vi "Graph-Init.vi"(8 "error in (no error)":errorcluster, 9 "SR830 in":refnum<vi>, 10 "Parameters":refnum<vi>, 11 "WaveformChart in":refnum<vi>) -> (0 "error out":errorcluster)   [LabVIEW 2016]
uses:
  controls/Parameters.ctl
  controls/Lambda.ctl
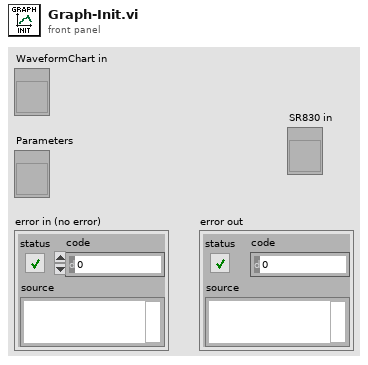
[diagram p1: front panel]
types:
  T1 = typedef "Parameters.ctl" = cluster{"Lambda":T2, "Power":dbl, "Frequency":dbl, "Stabilizing":dbl, "Samples":dbl, "File":path}
  T2 = typedef "Lambda.ctl" = cluster{"Init":dbl, "Final":dbl, "dx":dbl}
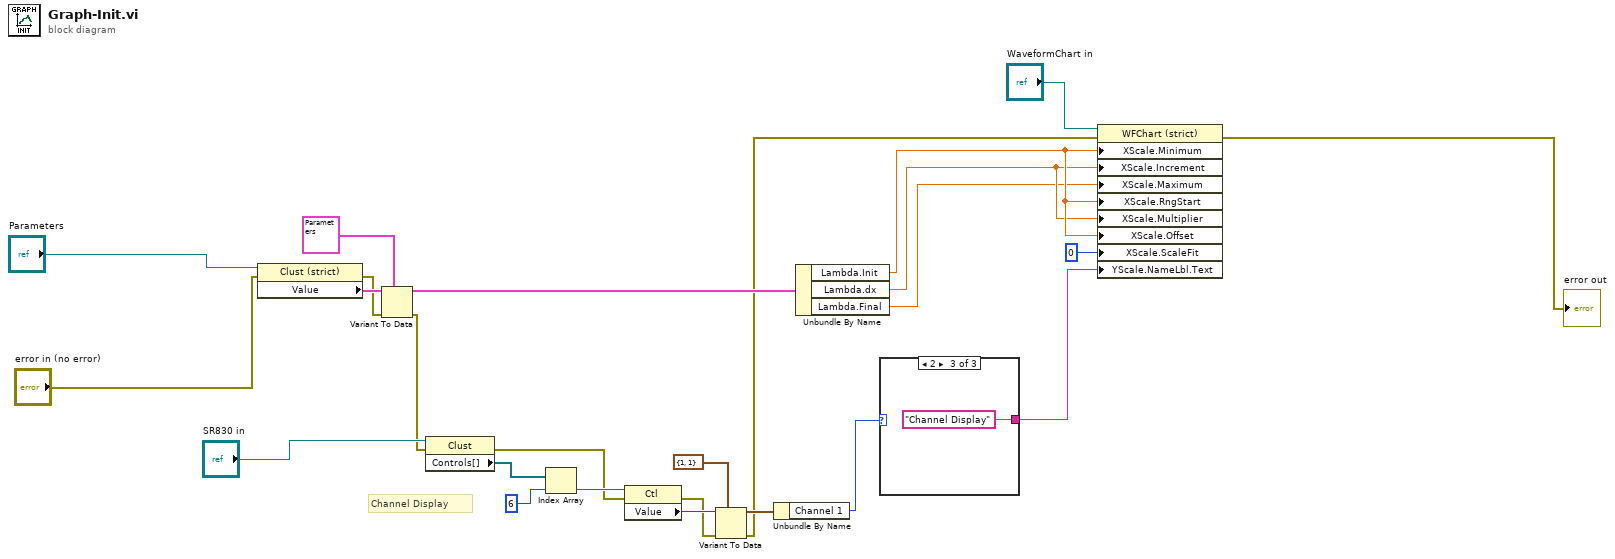
[diagram p0: block diagram]
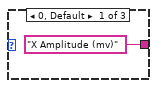
[diagram p2: hidden frame]
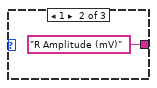
[diagram p3: hidden frame]
diagram:
  # "Channel Display"
  n1 = property class="Clust (strict)"(reference="Parameters", error in="error in (no error)") -> (error out=w15:errorcluster, "Value"=w16:T1)  [unwired: 1 out]
  n2 = Variant To Data(error in=w15, type=T1 {"Lambda"={"Init"=0.0, "Final"=0.0, "dx"=0.0}, "Power"=0.0, "Frequency"=0.0, "Stabilizing"=0.0, "Samples"=0.0, "File"=path ""} ("Parameters"), Variant=w16) -> (data=w18:T1, error out=w12:errorcluster)
  n3 = property class="Clust"(reference="SR830 in", error in=w12) -> (error out=w8:errorcluster, "Controls[]"=w11:refnum<vi>[])  [unwired: 1 out]
  n4 = Index Array(array=w11, index=6) -> (element=w9:refnum<vi>)
  n5 = property class="Ctl"(reference=w9, error in=w8) -> (error out=w6:errorcluster, "Value"=w7:variant)  [unwired: 1 out]
  n6 = Variant To Data(error in=w6, type=cluster{"Channel 1":u16, "Channel 2":u16} {"Channel 1"=1, "Channel 2"=1} ("Channel Display"), Variant=w7) -> (data=w4:cluster{"Channel 1":u16, "Channel 2":u16}, error out=w2:errorcluster)
  n7 = Unbundle By Name(w4) -> ("Channel 1"=w3:u16)
  n8 = Unbundle By Name(w18) -> ("Lambda.Init"=w23:dbl, "Lambda.dx"=w22:dbl, "Lambda.Final"=w21:dbl)
  n9 = case shown="2" w3 {
    tunnel: ["X Amplitude (mv)" "R Amplitude (mV)" "Channel Display"] -> w1
    frame 0, Default {
    }
    frame 1 {
    }
    frame 2 {
    }
  }
  n10 = property on="Property Node" class="WFChart (strict)"(reference="WaveformChart in", error in=w2, "XScale.Minimum"=w23, "XScale.Increment"=w22, "XScale.Maximum"=w21, "XScale.RngStart"=w23, "XScale.Multiplier"=w22, "XScale.Offset"=w23, "XScale.ScaleFit"=u8 0 ("X Scale.Scale Fit"), "YScale.NameLbl.Text"=w1) -> (error out=→"error out":errorcluster)  [unwired: 1 out]
